vi "Make Drink.vi"(8 "error in (no error)":errorcluster, 10 "Order Item in":refnum<class "Order Item.lvclass">, 11 "Barista in":refnum<class "Barista.lvclass">) -> (0 "error out":errorcluster, 2 "Order Item out":refnum<class "Order Item.lvclass">, 3 "Barista out":refnum<class "Barista.lvclass">)   [LabVIEW 2020, in "Barista.lvclass"]
uses:
  Barista.lvclass
  C:/Users/anton/Documents/GitHub/Triarc-Examples/Coffee Shop/Worker/Worker.lvclass
  Support/Order Item/Order Item.lvclass
  Worker/Worker.lvclass/Worker.ctl
  Person/Person.lvclass
  C:/Users/anton/Documents/GitHub/Triarc-Examples/Coffee Shop/Processes/People/Workers/Worker/Worker.lvclass
  C:/Users/anton/Documents/GitHub/Triarc-Examples/Coffee Shop/Processes/People/Person/Person.lvclass
  C:/Program Files (x86)/National Instruments/LabVIEW 2020/vi.lib/Asteme/Triarc Framework/View/View.lvclass
  C:/Program Files (x86)/National Instruments/LabVIEW 2020/vi.lib/Asteme/Triarc Framework/Process/Process.lvclass
  C:/Program Files (x86)/National Instruments/LabVIEW 2020/vi.lib/Asteme/Triarc Framework/Base/Base.lvclass
  C:/Program Files (x86)/National Instruments/LabVIEW 2020/vi.lib/Asteme/Triarc Framework/Error Handler Interface/Error Handler Interface.lvclass
  C:/Program Files (x86)/National Instruments/LabVIEW 2020/vi.lib/Asteme/Triarc Framework/Logging/Logging.lvclass
  C:/Users/anton/Documents/GitHub/Triarc-Examples/Coffee Shop/Processes/People/Process Job/Job Handler.lvclass
  C:/Users/anton/Documents/GitHub/Triarc-Examples/Coffee Shop/Processes/People/Workers/Barista/Barista.lvclass
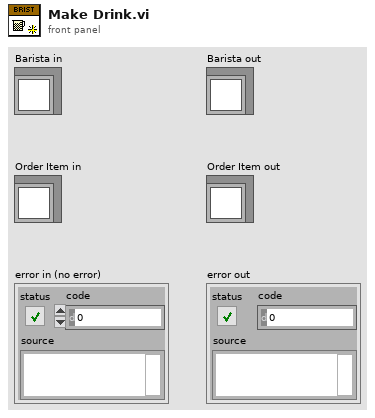
[diagram p1: front panel]
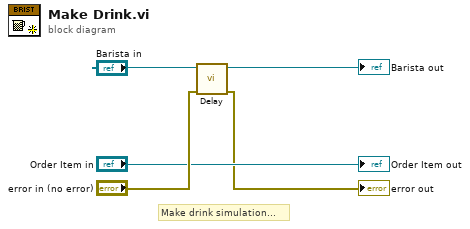
[diagram p0: block diagram]
diagram:
  # "Make drink simulation..."
  n1 = call "Delay.vi"("error in (no error)"="error in (no error)", "Person In"="Barista in") -> ("error out"=→"error out":errorcluster, "Person Out"=→"Barista out":refnum<class "Barista.lvclass">)  [unwired: 8 in]
  "Order Item out" <- "Order Item in"
